vi "Msg ListBox Append.vi"   [LabVIEW 2016, in "Common.lvlib"]
uses:
  <userlib>/Common Components/Common/Common.lvlib
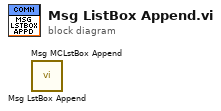
[diagram p0: block diagram]
diagram:
  n1 = call <userlib>:"Msg MCLstBox Append.vi"() -> ()  [unwired: 11 in, 1 out]
  n2 = call <userlib>:"Msg LstBox Append.vi"() -> ()  [unwired: 11 in, 1 out]
